vi "XY Graph 1-Normalize Multiple Plots.vi"(8 "error in (no error)":errorcluster, 10 "Selected Plots":i32[](array[numeric]), 11 "Selected Plot Info":T1) -> (0 "error out":errorcluster, 1 "1-Normalize Plot Message":string, 3 "Last 1-Normalized Plot":cluster{"t Array":dbl[], "IRF Array":dbl[]}, 4 "Single Plot?":bool)   [LabVIEW 2021, in "XY Graph Add-Ons.lvlib"]
uses:
  XY Graph Add-Ons.lvlib
  XY Graph Selected Plot Info.ctl
  XY Graph Refnum.ctl
  <vilib>/Utility/miscctls.llb/LVPoint32TypeDef.ctl
  Strings/Strings.lvlib
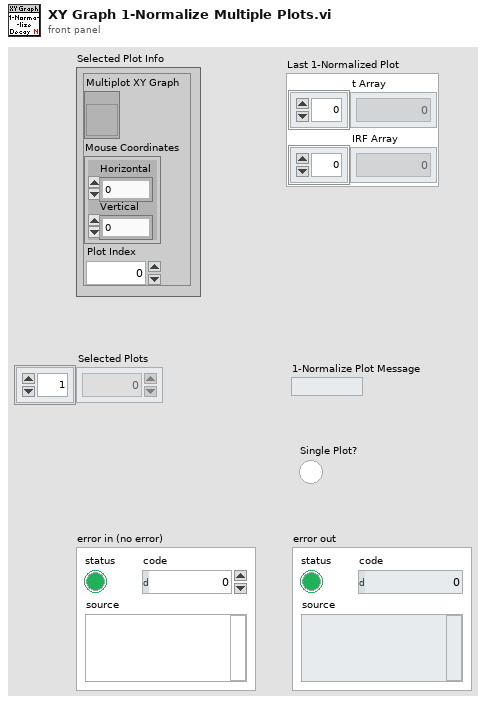
[diagram p1: front panel]
types:
  T1 = typedef "XY Graph Add-Ons.lvlib/XY Graph Selected Plot Info.ctl" = cluster{"Multiplot XY Graph":T2, "Mouse Coordinates":T3, "Plot Index":i32}
  T2 = typedef "XY Graph Add-Ons.lvlib/XY Graph Refnum.ctl" = refnum<vi>
  T3 = typedef "LVPoint32TypeDef.ctl" = cluster{"Horizontal":i32, "Vertical":i32}
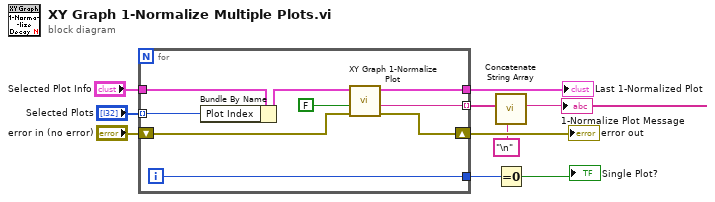
[diagram p0: block diagram]
diagram:
  n1 = for {
    tunnel: "Selected Plot Info" -> [w18]
    tunnel: [w17] -> w8 mode=indexing
    tunnel: [w15] -> w6
    shift-right: [w16] -> w7
    shift-left: "error in (no error)" -> [w19]
    tunnel: "Selected Plots" -> [w13] mode=indexing
    tunnel: [w12] -> w2
    i -> [w12]
    n2 = Bundle By Name(cluster=w18, "Plot Index"=w13) -> (w14:T1)
    n3 = call "XY Graph 1-Normalize Plot.vi"("error in (no error)"=w19, "Replace Plot (T)?"=FALSE, "Selected Plot Info"=w14) -> ("Error Out"=w16:errorcluster, "1-Normalize Plot Message"=w17:string, "1-Normalized Plot"=w15:cluster{"t Array":dbl[], "IRF Array":dbl[]})  [unwired: 6 in]
  }
  "error out" <- w7
  "Last 1-Normalized Plot" <- w6
  n4 = call "Concatenate String Array.vi"("Separator (TAB)"="\n", "String Array"=w8) -> ("Formatted String"=→"1-Normalize Plot Message":string)  [unwired: 9 in]
  n5 = Equal To 0?(x=w2) -> (x = 0?=→"Single Plot?":bool)
